vi "MAC Address.vi"(8 "error out":errorcluster, 11 "VISA resource name":refnum<visa-resource-name>) -> (0 "error out":errorcluster, 2 "Ethernet MAC address":string, 3 "VISA resource name out":refnum<visa-resource-name>, 4 "Device Errors":cluster{"code":i32, "Text":string}[](array[cluster]))   [LabVIEW 2014, in "Stanford Research DG645 - Driver.lvlib"]
doc: "Interface Command: EMAC?\nInstrument Error Check\n\nQuery the DG645's Ethernet MAC address."
uses:
  Stanford Research DG645 - Driver.lvlib
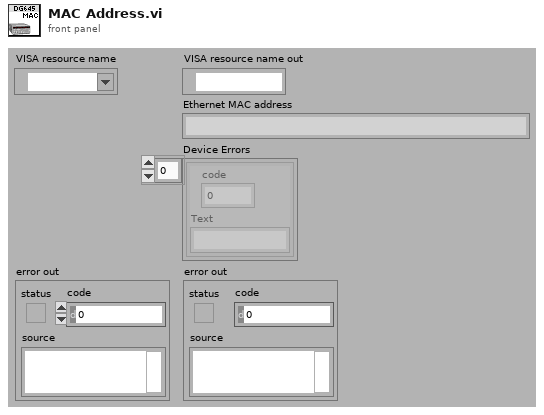
[diagram p1: front panel]
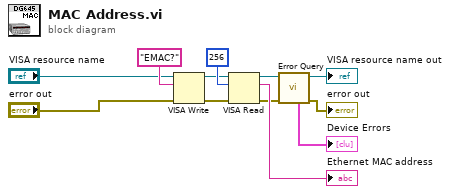
[diagram p0: block diagram]
diagram:
  n1 = VISA Write(VISA resource name="VISA resource name", write buffer="EMAC?" ("ID Query"), error in (no error)="error out") -> (VISA resource name out=w9:refnum<visa-resource-name>, error out=w10:errorcluster)  [unwired: 1 out]
  n2 = VISA Read(VISA resource name=w9, byte count=u32 256, error in (no error)=w10) -> (VISA resource name out=w8:refnum<visa-resource-name>, read buffer=→"Ethernet MAC address":string, error out=w1:errorcluster)  [unwired: 1 out]
  n3 = call "Error Query.vi"("error in (no error)"=w1, "VISA resource name"=w8) -> ("error out"=→"error out":errorcluster, "VISA resource name out"=→"VISA resource name out":refnum<visa-resource-name>, "Device Errors"=→"Device Errors":cluster{"code":i32, "Text":string}[])  [unwired: 7 in]
